vi "certaintyGraph Computer Ver.vi"() -> ()   [LabVIEW 2012]
panel:
  out "Intensity Graph":i16[][](graph)
  in  "Wait":i32
  in  "Degrees":dbl
  in  "distance front":fxp<+/-,64,32>
  in  "stop":bool
  in  "Sensor x":i16
  in  "Sensor y":i16
  in  "distance right":fxp<+/-,64,32>
  in  "distance left":fxp<+/-,64,32>
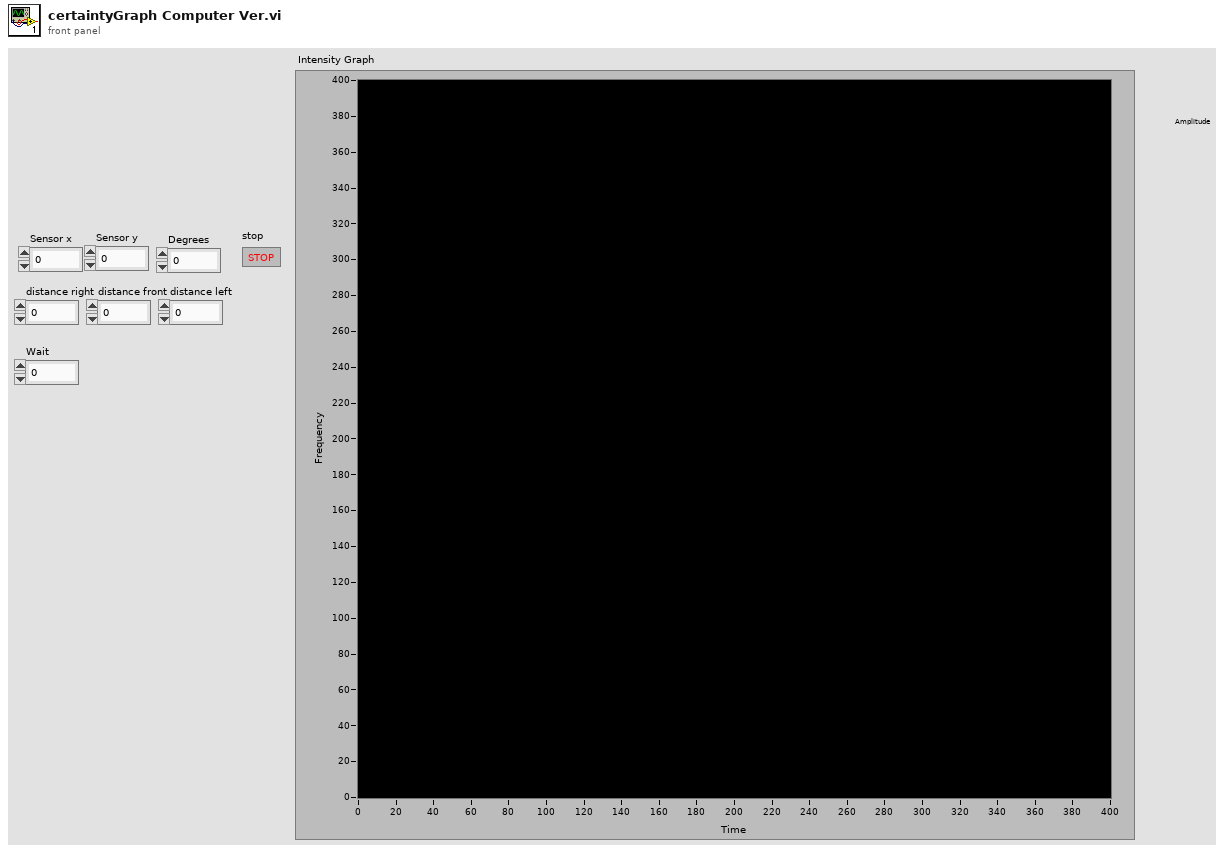
[diagram p1: front panel]
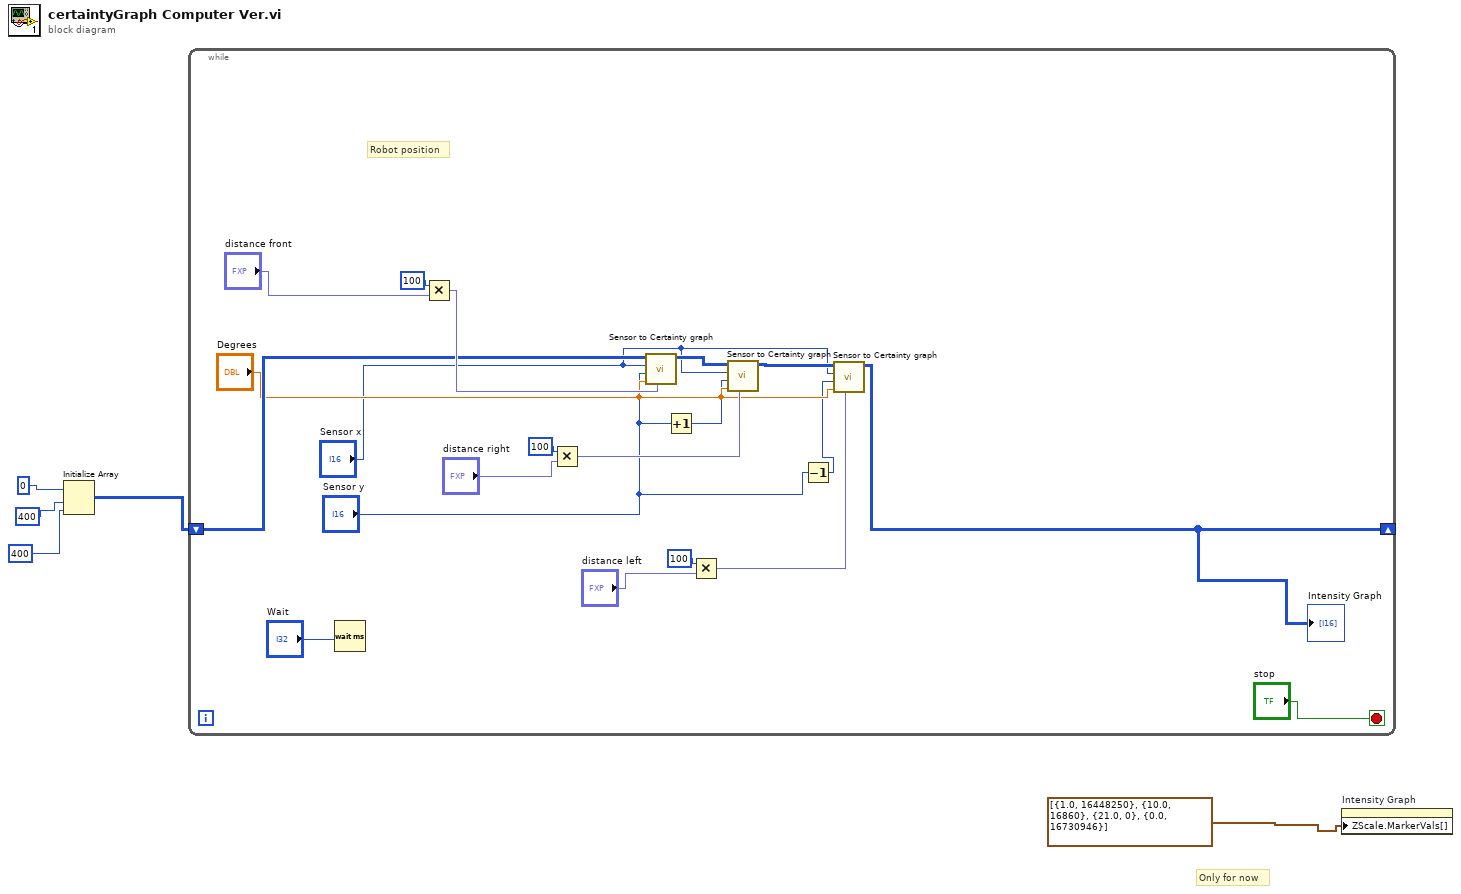
[diagram p0: block diagram]
diagram:
  # "Only for now"
  n1 = Initialize Array(i16 0, i16 400, 400) -> (w3:i16[][])
  n2 = while {
    shift-right: [w6] -> _
    shift-left: w3 -> [w22]
    stop <- "stop" stop-if-true
    # "Robot position"
    n3 = Wait (ms)(milliseconds to wait="Wait") -> ()  [unwired: 1 out]
    n4 = Multiply(x=100, y="distance front") -> (x*y=w23:fxp<+/-,64,64>)
    n5 = Multiply(x=100, y="distance right") -> (x*y=w20:fxp<+/-,64,64>)
    n6 = call "Sensor to Certainty graph.vi"("Distance"=w23, "Degrees"="Degrees", "Sensor y"="Sensor y", "Sensor x"="Sensor x", "Array 2"=w22) -> ("Array 3"=w19:i16[][])  [unwired: 6 in]
    n7 = Increment(x="Sensor y") -> (x+1=w16:i16)
    n8 = Multiply(x=100, y="distance left") -> (x*y=w11:fxp<+/-,64,64>)
    n9 = call "Sensor to Certainty graph.vi"("Distance"=w20, "Degrees"="Degrees", "Sensor y"=w16, "Sensor x"="Sensor x", "Array 2"=w19) -> ("Array 3"=w18:i16[][])  [unwired: 6 in]
    n10 = Decrement(x="Sensor y") -> (x-1=w14:i16)
    n11 = call "Sensor to Certainty graph.vi"("Distance"=w11, "Degrees"="Degrees", "Sensor y"=w14, "Sensor x"="Sensor x", "Array 2"=w18) -> ("Array 3"=w6:i16[][])  [unwired: 6 in]
    "Intensity Graph" <- w6
  }
  n12 = property on="Intensity Graph" class="IntGraph (strict)"("ZScale.MarkerVals[]"=cluster{dbl, u32}[] [{1.0, 16448250}, {10.0, 16860}, {21.0, 0}, {0.0, 16730946}] ("Z Scale.Marker Values[]")) -> ()  [unwired: 2 in, 2 out]
